vi "Set SG Path.vi"(0 "Scalar SG Si2250 Path in":refnum<class "SG SC2250 Path.lvclass">, 5 "Cal point in":T1, 11 "error in (no error)":errorcluster) -> (4 "Scalar SG Si2250 Path out":refnum<class "SG SC2250 Path.lvclass">, 6 "Cal point out":T1, 8 "Source Gain":dbl, 10 "Digital Gain":dbl, 15 "error out":errorcluster)   [LabVIEW 2023, in "RFFixtureCharact.RFPM.lvlib" / "SG SC2250 Path.lvclass"]
uses:
  SG SC2250 Path.lvclass
  C:/srd-semi-rfcal-software/AuxTools/STSRFFixtureCharactUtility/Source/Code Modules/Common/Base Classes/Path/Path.lvclass
  C:/srd-semi-rfcal-software/AuxTools/STSRFFixtureCharactUtility/Source/Code Modules/Fixture/RFPM/Scalar/Paths/SG Path/SG 18GHz Path.lvclass
  Public/Base Classes/Scalar/Scalar Path/Type Definitions/Cal Point.ctl
  <instrlib>/niRFPM/niRFPM.llb/NI-RFPM Set TX Path By Switch Path String.vi
  Public/Base Classes/Scalar/Scalar Path/Scalar Path.lvclass
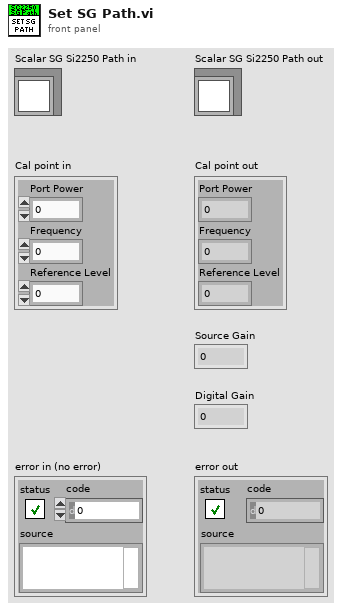
[diagram p1: front panel]
types:
  T1 = typedef "RFFixtureCharact.Public.lvlib/Scalar Path.lvclass/Cal Point.ctl" = cluster{"Port Power":dbl, "Frequency":dbl, "Reference Level":dbl}
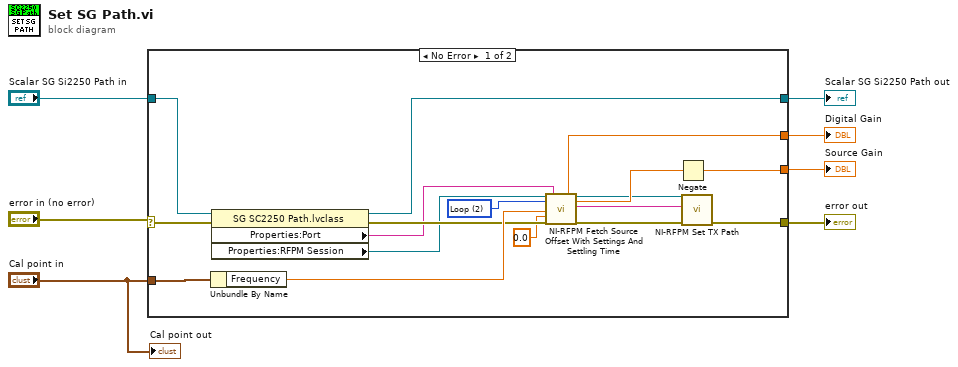
[diagram p0: block diagram]
diagram:
  n1 = case shown="No Error" "error in (no error)" {
    selector: "error in (no error)" -> [w16 w26]
    tunnel: [w17 w26] -> w7
    tunnel: [w14 w25] -> w5
    tunnel: "Scalar SG Si2250 Path in" -> [w15 w25]
    tunnel: [w18 _] -> w6
    tunnel: "Cal point in" -> [w9 _]
    tunnel: [w8 _] -> w2
    frame No Error {
      w11 = u32 2 items=["Unspecified"=3, "Direct"=0, "Gain"=1, "Loop"=2, "Two Tone"=4] ("Source Path")
      n2 = Unbundle By Name(w9) -> ("Frequency"=w24:dbl)
      n3 = property class="SG SC2250 Path.lvclass"(reference=w15, error in=w16) -> (reference out=w14:refnum<class "SG SC2250 Path.lvclass">, error out=w23:errorcluster, "Properties:Port"=w13:string, "Properties:RFPM Session"=w12:refnum<k15>)
      n4 = call <instrlib>:"NI-RFPM Fetch Source Offset With Settings And Settling Time.vi"("instrument handle"=w12, "Source Path"=w11, "Frequency"=w24, "Power"=0.0, "error in"=w23, "Port"=w13) -> ("Digital Gain"=w8:dbl, "instrument handle out"=w19:refnum<k15>, "Source Offset"=w22:dbl, "Switch Path String"=w21:string, "error out"=w20:errorcluster)  [unwired: 7 in, 2 out]
      n5 = Negate(x=w22) -> (-x=w18:dbl)
      n6 = call-poly <instrlib>:"NI-RFPM Set TX Path.vi"("instrument handle"=w19, "TX Switch Path"=w21, "error in (no error)"=w20) -> ("error out"=w17:errorcluster)  [unwired: 11 in, 1 out]
    }
    frame Error {
    }
  }
  "error out" <- w7
  "Scalar SG Si2250 Path out" <- w5
  "Source Gain" <- w6
  "Digital Gain" <- w2
  "Cal point out" <- "Cal point in"
